vi "RFSG Generate Signal.vi"(8 "error in (no error)":errorcluster, 9 "input IQ rate":dbl=100000000.0 format="%#_6p", 10 "Samples Per Cycle":i32, 11 "RFSG Reference In":refnum<k15>) -> (0 "error out":errorcluster, 3 "RFSG Reference Out":refnum<k15>)   [LabVIEW 2021]
uses:
  <instrlib>/niRFSG/niRFSGExamplesSupport.llb/rfsg_Resample and Write (I-Q).vi
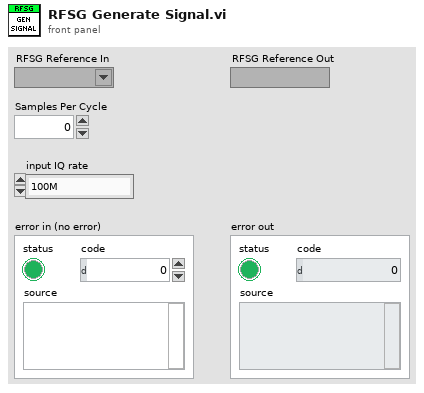
[diagram p1: front panel]
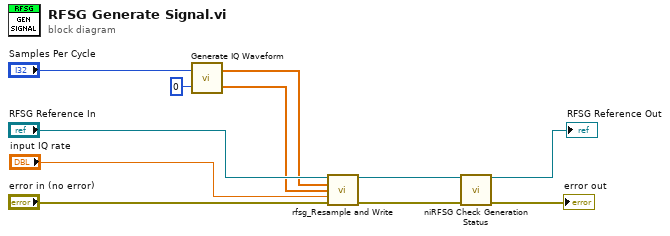
[diagram p0: block diagram]
diagram:
  n1 = call "Generate IQ Waveform.vi"("Selected Waveform"=u16 0, "Samples Per Cycle"="Samples Per Cycle") -> ("Q"=w2:dbl[], "I"=w3:dbl[])
  n2 = call-poly <instrlib>:"rfsg_Resample and Write.vi"("instrument handle in"="RFSG Reference In", "I"=w3, "Q"=w2, "input IQ rate"="input IQ rate", "error in"="error in (no error)") -> ("instrument handle out"=w6:refnum<k15>, "error out"=w4:errorcluster)  [unwired: 8 in, 1 out]
  n3 = call <instrlib>:"niRFSG Check Generation Status.vi"("instrument handle"=w6, "error in"=w4) -> ("instrument handle out"=→"RFSG Reference Out":refnum<k15>, "error out"=→"error out":errorcluster)  [unwired: 11 in, 1 out]
